vi "CRYAdd Global Buffer.vi"(9 "Gen Idx":u32, 11 "Data":sgl[](array[numeric])) -> ()   [LabVIEW 2013]
uses:
  CRYMisc vis settings global.vi
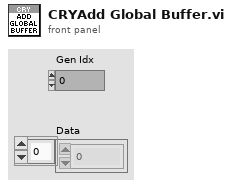
[diagram p1: front panel]
types:
  T1 = cluster{"Gen Idx":i32, "Chn Idx":i32, "Data":sgl[]}[]
  T2 = cluster{"Gen Idx":i32, "Chn Idx":i32, "Data":sgl[]}
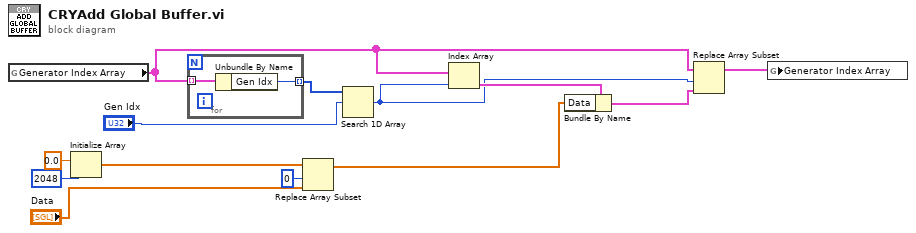
[diagram p0: block diagram]
diagram:
  n1 = global read "CRYMisc vis settings global.vi" "Generator Index Array"() -> (w3:T1)
  n2 = Initialize Array(sgl 0.0 ("element"), 2048 ("dimension size")) -> (w9:sgl[])
  n3 = for {
    tunnel: w3 -> [w15] mode=indexing
    tunnel: [w14] -> w8 mode=indexing
    n4 = Unbundle By Name(w15) -> ("Gen Idx"=w14:i32)
  }
  n5 = Replace Array Subset(array=w9, new element="Data", index=0) -> (w5:sgl[])
  n6 = Search 1D Array(1D array=w8, element="Gen Idx") -> (index of element=w2:i32)  [unwired: 1 in]
  n7 = Index Array(array=w3, index=w2) -> (element=w6:T2)
  n8 = Bundle By Name(cluster=w6, "Data"=w5) -> (w4:T2)
  n9 = Replace Array Subset(array=w3, new element=w4, index=w2) -> (w1:T1)
  n10 = global write "CRYMisc vis settings global.vi" "Generator Index Array"(w1) -> ()
